vi "CAN Jaguar Set PID.vi"(0 "CAN Jaguar Ref":T1={"Device Number"=0, "Control Mode"=enum."Percent VBus", "Inverted"=FALSE, "Semaphore"=refnum, "Max Vout"=12.0, "DevStatus"={"status"=FALSE, "code"=0, "source"=""}}, 5 "P":dbl, 7 "I":dbl, 9 "D":dbl, 11 "error in (no error)":errorcluster) -> (4 "CAN Jaguar Ref Out":T1={"Device Number"=0, "Control Mode"=enum."Percent VBus", "Inverted"=FALSE, "Semaphore"=refnum, "Max Vout"=12.0, "DevStatus"={"status"=FALSE, "code"=0, "source"=""}}, 15 "error out":errorcluster)   [LabVIEW 2009, in "CAN.lvlib"]
uses:
  CAN.lvlib
  SubVIs/CAN Motor Message IDs.ctl
  SubVIs/CAN Jaguar Control Mode.ctl
  SubVIs/CAN Jaguar Ref.ctl
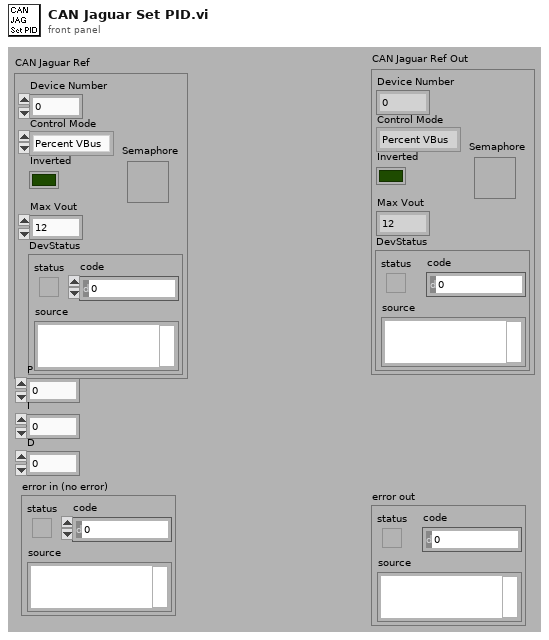
[diagram p1: front panel]
types:
  T1 = typedef "CAN.lvlib/CAN Jaguar Ref.ctl" = cluster{"Device Number":u8, "Control Mode":T2, "Inverted":bool, "Semaphore":T3, "Max Vout":dbl, "DevStatus":errorcluster}
  T2 = typedef "CAN.lvlib/CAN Jaguar Control Mode.ctl" = enum16{"Percent VBus", "Speed", "Position", "Current"}
  T3 = typedef "Semaphore RefNum" = refnum<k1>
  T4 = enum16{"big-endian, network order", "native, host order", "little-endian"}
  T5 = typedef "CAN.lvlib/CAN Motor Message IDs.ctl" = u32
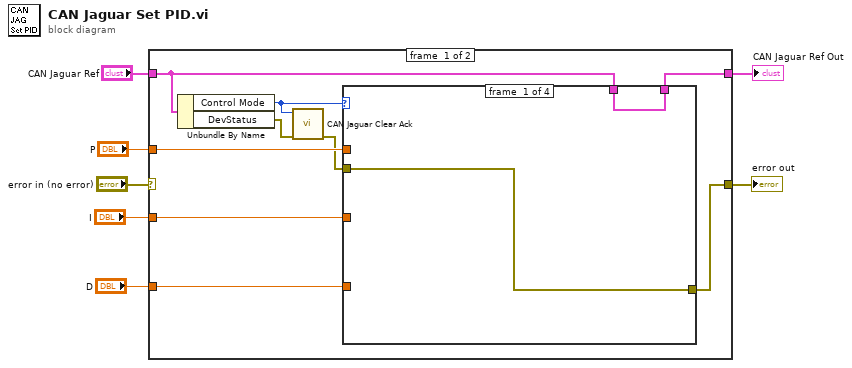
[diagram p0: block diagram]
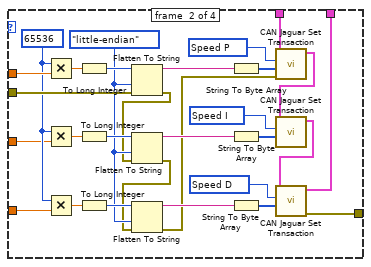
[diagram p2: hidden frame]
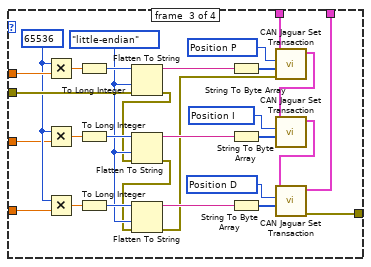
[diagram p3: hidden frame]
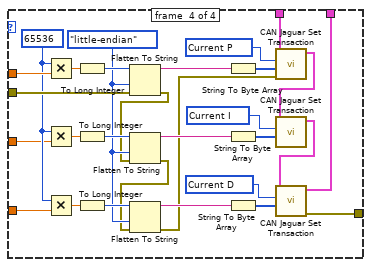
[diagram p4: hidden frame]
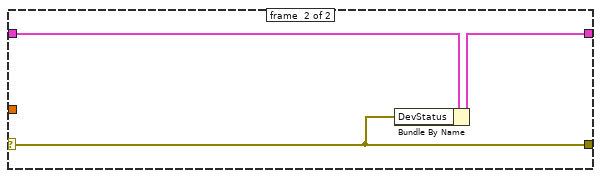
[diagram p5: hidden frame]
diagram:
  n1 = case shown="No Error" "error in (no error)" {
    selector: "error in (no error)" -> [_ w106]
    tunnel: [w13 w106] -> w7
    tunnel: [w8 w107] -> w5
    tunnel: "CAN Jaguar Ref" -> [w9 w108]
    tunnel: "P" -> [w16 _]
    tunnel: "D" -> [w15 _]
    tunnel: "I" -> [w14 _]
    frame #0 {
      n2 = Unbundle By Name(w9) -> ("Control Mode"=w10:T2, "DevStatus"=w12:errorcluster)
      n3 = call "CAN Jaguar Clear Ack.vi"("DevStatus"=w12, "Device Number"=w10) -> ("error out"=w11:errorcluster)  [unwired: 9 out]
      n4 = case shown="\"Speed\"" w10 {
        tunnel: w11 -> [w18 w46 w75 w104]
        tunnel: w16 -> [_ w44 w73 w102]
        tunnel: w15 -> [_ w34 w63 w92]
        tunnel: w14 -> [_ w33 w62 w91]
        tunnel: [w18 w20 w49 w77] -> w13
        tunnel: w9 -> [w17 w29 w56 w86]
        tunnel: [w17 w19 w48 w82] -> w8
        frame #0 {
        }
        frame #1 {
          w36 = T4."little-endian" ("byte order (0:big-endian, network order)")
          w30 = T5 33686848 items=["Volt Enable"=33685504, "Volt Disable"=33685568, "Volt Set"=33685632, "Volt Set Ramp"=33685696, "Speed Enable"=33686528, "Speed Disable"=33686592, "Speed Set"=33686656, "Speed P"=33686720, "Speed I"=33686784, "Speed D"=33686848, "Speed Ref"=33686912, "Position Enable"=33688576, "Position Disable"=33688640, "Position Set"=33688704, "Position P"=33688768, "Position I"=33688832, "Position D"=33688896, "Position Ref"=33688960, "Current Enable"=33689600, "Current Disable"=33689664, "Current Set"=33689728, "Current P"=33689792, "Current I"=33689856, "Current D"=33689920, "Status VOut"=33690624, "Status VBus"=33690688, "Status Current"=33690752, "Status Temp"=33690816, "Status Position"=33690880, "Status Speed"=33690944, "Status Limit"=33691008, "Status Fault"=33691072, "Status Power"=33691136, "Config Num Brushes"=33692672, "Config Encoder Lines"=33692736, "Config Pot Turns"=33692800, "Config Brake Coast"=33692864, "Config Limit Mode"=33692928, "Config Limit Fwd"=33692992, "Config Limit Rev"=33693056, "Config Max VOut"=33693120, "Config Fault Time"=33693184, "Motor Ack"=33693696] ("CAN Motor Message IDs")
          w24 = T5 33686784 items=["Volt Enable"=33685504, "Volt Disable"=33685568, "Volt Set"=33685632, "Volt Set Ramp"=33685696, "Speed Enable"=33686528, "Speed Disable"=33686592, "Speed Set"=33686656, "Speed P"=33686720, "Speed I"=33686784, "Speed D"=33686848, "Speed Ref"=33686912, "Position Enable"=33688576, "Position Disable"=33688640, "Position Set"=33688704, "Position P"=33688768, "Position I"=33688832, "Position D"=33688896, "Position Ref"=33688960, "Current Enable"=33689600, "Current Disable"=33689664, "Current Set"=33689728, "Current P"=33689792, "Current I"=33689856, "Current D"=33689920, "Status VOut"=33690624, "Status VBus"=33690688, "Status Current"=33690752, "Status Temp"=33690816, "Status Position"=33690880, "Status Speed"=33690944, "Status Limit"=33691008, "Status Fault"=33691072, "Status Power"=33691136, "Config Num Brushes"=33692672, "Config Encoder Lines"=33692736, "Config Pot Turns"=33692800, "Config Brake Coast"=33692864, "Config Limit Mode"=33692928, "Config Limit Fwd"=33692992, "Config Limit Rev"=33693056, "Config Max VOut"=33693120, "Config Fault Time"=33693184, "Motor Ack"=33693696] ("CAN Motor Message IDs")
          w35 = 65536
          w27 = T5 33686720 items=["Volt Enable"=33685504, "Volt Disable"=33685568, "Volt Set"=33685632, "Volt Set Ramp"=33685696, "Speed Enable"=33686528, "Speed Disable"=33686592, "Speed Set"=33686656, "Speed P"=33686720, "Speed I"=33686784, "Speed D"=33686848, "Speed Ref"=33686912, "Position Enable"=33688576, "Position Disable"=33688640, "Position Set"=33688704, "Position P"=33688768, "Position I"=33688832, "Position D"=33688896, "Position Ref"=33688960, "Current Enable"=33689600, "Current Disable"=33689664, "Current Set"=33689728, "Current P"=33689792, "Current I"=33689856, "Current D"=33689920, "Status VOut"=33690624, "Status VBus"=33690688, "Status Current"=33690752, "Status Temp"=33690816, "Status Position"=33690880, "Status Speed"=33690944, "Status Limit"=33691008, "Status Fault"=33691072, "Status Power"=33691136, "Config Num Brushes"=33692672, "Config Encoder Lines"=33692736, "Config Pot Turns"=33692800, "Config Brake Coast"=33692864, "Config Limit Mode"=33692928, "Config Limit Fwd"=33692992, "Config Limit Rev"=33693056, "Config Max VOut"=33693120, "Config Fault Time"=33693184, "Motor Ack"=33693696] ("CAN Motor Message IDs")
          n5 = Multiply(x=w35, y=w44) -> (x*y=w45:dbl)
          n6 = Multiply(x=w35, y=w33) -> (x*y=w43:dbl)
          n7 = Multiply(x=w35, y=w34) -> (x*y=w40:dbl)
          n8 = To Long Integer(number=w45) -> (32bit integer=w47:i32)
          n9 = To Long Integer(number=w43) -> (32bit integer=w42:i32)
          n10 = To Long Integer(number=w40) -> (32bit integer=w41:i32)
          n11 = Flatten To String(anything=w47, byte order (0:big-endian, network order)=w36, error in (no error)=w46) -> (data string=w39:string, error out=w32:errorcluster)  [unwired: 2 out]
          n12 = Flatten To String(anything=w42, byte order (0:big-endian, network order)=w36, error in (no error)=w32) -> (data string=w38:string, error out=w31:errorcluster)  [unwired: 2 out]
          n13 = Flatten To String(anything=w41, byte order (0:big-endian, network order)=w36, error in (no error)=w31) -> (data string=w37:string, error out=w28:errorcluster)  [unwired: 2 out]
          n14 = String To Byte Array(string=w39) -> (unsigned byte array=w26:u8[])
          n15 = String To Byte Array(string=w38) -> (unsigned byte array=w25:u8[])
          n16 = String To Byte Array(string=w37) -> (unsigned byte array=w22:u8[])
          n17 = call "CAN Jaguar Set Transaction.vi"("error in"=w28, "Data"=w26, "Message ID"=w27, "CAN Jaguar Ref"=w29) -> ("CAN Jaguar Ref Out"=w23:T1)  [unwired: 7 out]
          n18 = call "CAN Jaguar Set Transaction.vi"("Data"=w25, "Message ID"=w24, "CAN Jaguar Ref"=w23) -> ("CAN Jaguar Ref Out"=w21:T1)  [unwired: 1 in, 7 out]
          n19 = call "CAN Jaguar Set Transaction.vi"("Data"=w22, "Message ID"=w30, "CAN Jaguar Ref"=w21) -> ("error out"=w20:errorcluster, "CAN Jaguar Ref Out"=w19:T1)  [unwired: 1 in, 6 out]
        }
        frame #2 {
          w65 = T4."little-endian" ("byte order (0:big-endian, network order)")
          w53 = T5 33688896 items=["Volt Enable"=33685504, "Volt Disable"=33685568, "Volt Set"=33685632, "Volt Set Ramp"=33685696, "Speed Enable"=33686528, "Speed Disable"=33686592, "Speed Set"=33686656, "Speed P"=33686720, "Speed I"=33686784, "Speed D"=33686848, "Speed Ref"=33686912, "Position Enable"=33688576, "Position Disable"=33688640, "Position Set"=33688704, "Position P"=33688768, "Position I"=33688832, "Position D"=33688896, "Position Ref"=33688960, "Current Enable"=33689600, "Current Disable"=33689664, "Current Set"=33689728, "Current P"=33689792, "Current I"=33689856, "Current D"=33689920, "Status VOut"=33690624, "Status VBus"=33690688, "Status Current"=33690752, "Status Temp"=33690816, "Status Position"=33690880, "Status Speed"=33690944, "Status Limit"=33691008, "Status Fault"=33691072, "Status Power"=33691136, "Config Num Brushes"=33692672, "Config Encoder Lines"=33692736, "Config Pot Turns"=33692800, "Config Brake Coast"=33692864, "Config Limit Mode"=33692928, "Config Limit Fwd"=33692992, "Config Limit Rev"=33693056, "Config Max VOut"=33693120, "Config Fault Time"=33693184, "Motor Ack"=33693696] ("CAN Motor Message IDs")
          w52 = T5 33688832 items=["Volt Enable"=33685504, "Volt Disable"=33685568, "Volt Set"=33685632, "Volt Set Ramp"=33685696, "Speed Enable"=33686528, "Speed Disable"=33686592, "Speed Set"=33686656, "Speed P"=33686720, "Speed I"=33686784, "Speed D"=33686848, "Speed Ref"=33686912, "Position Enable"=33688576, "Position Disable"=33688640, "Position Set"=33688704, "Position P"=33688768, "Position I"=33688832, "Position D"=33688896, "Position Ref"=33688960, "Current Enable"=33689600, "Current Disable"=33689664, "Current Set"=33689728, "Current P"=33689792, "Current I"=33689856, "Current D"=33689920, "Status VOut"=33690624, "Status VBus"=33690688, "Status Current"=33690752, "Status Temp"=33690816, "Status Position"=33690880, "Status Speed"=33690944, "Status Limit"=33691008, "Status Fault"=33691072, "Status Power"=33691136, "Config Num Brushes"=33692672, "Config Encoder Lines"=33692736, "Config Pot Turns"=33692800, "Config Brake Coast"=33692864, "Config Limit Mode"=33692928, "Config Limit Fwd"=33692992, "Config Limit Rev"=33693056, "Config Max VOut"=33693120, "Config Fault Time"=33693184, "Motor Ack"=33693696] ("CAN Motor Message IDs")
          w64 = 65536
          w57 = T5 33688768 items=["Volt Enable"=33685504, "Volt Disable"=33685568, "Volt Set"=33685632, "Volt Set Ramp"=33685696, "Speed Enable"=33686528, "Speed Disable"=33686592, "Speed Set"=33686656, "Speed P"=33686720, "Speed I"=33686784, "Speed D"=33686848, "Speed Ref"=33686912, "Position Enable"=33688576, "Position Disable"=33688640, "Position Set"=33688704, "Position P"=33688768, "Position I"=33688832, "Position D"=33688896, "Position Ref"=33688960, "Current Enable"=33689600, "Current Disable"=33689664, "Current Set"=33689728, "Current P"=33689792, "Current I"=33689856, "Current D"=33689920, "Status VOut"=33690624, "Status VBus"=33690688, "Status Current"=33690752, "Status Temp"=33690816, "Status Position"=33690880, "Status Speed"=33690944, "Status Limit"=33691008, "Status Fault"=33691072, "Status Power"=33691136, "Config Num Brushes"=33692672, "Config Encoder Lines"=33692736, "Config Pot Turns"=33692800, "Config Brake Coast"=33692864, "Config Limit Mode"=33692928, "Config Limit Fwd"=33692992, "Config Limit Rev"=33693056, "Config Max VOut"=33693120, "Config Fault Time"=33693184, "Motor Ack"=33693696] ("CAN Motor Message IDs")
          n20 = Multiply(x=w64, y=w73) -> (x*y=w74:dbl)
          n21 = Multiply(x=w64, y=w62) -> (x*y=w72:dbl)
          n22 = Multiply(x=w64, y=w63) -> (x*y=w69:dbl)
          n23 = To Long Integer(number=w74) -> (32bit integer=w76:i32)
          n24 = To Long Integer(number=w72) -> (32bit integer=w71:i32)
          n25 = To Long Integer(number=w69) -> (32bit integer=w70:i32)
          n26 = Flatten To String(anything=w76, byte order (0:big-endian, network order)=w65, error in (no error)=w75) -> (data string=w68:string, error out=w61:errorcluster)  [unwired: 2 out]
          n27 = Flatten To String(anything=w71, byte order (0:big-endian, network order)=w65, error in (no error)=w61) -> (data string=w67:string, error out=w60:errorcluster)  [unwired: 2 out]
          n28 = Flatten To String(anything=w70, byte order (0:big-endian, network order)=w65, error in (no error)=w60) -> (data string=w66:string, error out=w58:errorcluster)  [unwired: 2 out]
          n29 = String To Byte Array(string=w68) -> (unsigned byte array=w59:u8[])
          n30 = String To Byte Array(string=w67) -> (unsigned byte array=w55:u8[])
          n31 = String To Byte Array(string=w66) -> (unsigned byte array=w54:u8[])
          n32 = call "CAN Jaguar Set Transaction.vi"("error in"=w58, "Data"=w59, "Message ID"=w57, "CAN Jaguar Ref"=w56) -> ("CAN Jaguar Ref Out"=w51:T1)  [unwired: 7 out]
          n33 = call "CAN Jaguar Set Transaction.vi"("Data"=w55, "Message ID"=w52, "CAN Jaguar Ref"=w51) -> ("CAN Jaguar Ref Out"=w50:T1)  [unwired: 1 in, 7 out]
          n34 = call "CAN Jaguar Set Transaction.vi"("Data"=w54, "Message ID"=w53, "CAN Jaguar Ref"=w50) -> ("error out"=w49:errorcluster, "CAN Jaguar Ref Out"=w48:T1)  [unwired: 1 in, 6 out]
        }
        frame #3 {
          w94 = T4."little-endian" ("byte order (0:big-endian, network order)")
          w81 = T5 33689920 items=["Volt Enable"=33685504, "Volt Disable"=33685568, "Volt Set"=33685632, "Volt Set Ramp"=33685696, "Speed Enable"=33686528, "Speed Disable"=33686592, "Speed Set"=33686656, "Speed P"=33686720, "Speed I"=33686784, "Speed D"=33686848, "Speed Ref"=33686912, "Position Enable"=33688576, "Position Disable"=33688640, "Position Set"=33688704, "Position P"=33688768, "Position I"=33688832, "Position D"=33688896, "Position Ref"=33688960, "Current Enable"=33689600, "Current Disable"=33689664, "Current Set"=33689728, "Current P"=33689792, "Current I"=33689856, "Current D"=33689920, "Status VOut"=33690624, "Status VBus"=33690688, "Status Current"=33690752, "Status Temp"=33690816, "Status Position"=33690880, "Status Speed"=33690944, "Status Limit"=33691008, "Status Fault"=33691072, "Status Power"=33691136, "Config Num Brushes"=33692672, "Config Encoder Lines"=33692736, "Config Pot Turns"=33692800, "Config Brake Coast"=33692864, "Config Limit Mode"=33692928, "Config Limit Fwd"=33692992, "Config Limit Rev"=33693056, "Config Max VOut"=33693120, "Config Fault Time"=33693184, "Motor Ack"=33693696] ("CAN Motor Message IDs")
          w80 = T5 33689856 items=["Volt Enable"=33685504, "Volt Disable"=33685568, "Volt Set"=33685632, "Volt Set Ramp"=33685696, "Speed Enable"=33686528, "Speed Disable"=33686592, "Speed Set"=33686656, "Speed P"=33686720, "Speed I"=33686784, "Speed D"=33686848, "Speed Ref"=33686912, "Position Enable"=33688576, "Position Disable"=33688640, "Position Set"=33688704, "Position P"=33688768, "Position I"=33688832, "Position D"=33688896, "Position Ref"=33688960, "Current Enable"=33689600, "Current Disable"=33689664, "Current Set"=33689728, "Current P"=33689792, "Current I"=33689856, "Current D"=33689920, "Status VOut"=33690624, "Status VBus"=33690688, "Status Current"=33690752, "Status Temp"=33690816, "Status Position"=33690880, "Status Speed"=33690944, "Status Limit"=33691008, "Status Fault"=33691072, "Status Power"=33691136, "Config Num Brushes"=33692672, "Config Encoder Lines"=33692736, "Config Pot Turns"=33692800, "Config Brake Coast"=33692864, "Config Limit Mode"=33692928, "Config Limit Fwd"=33692992, "Config Limit Rev"=33693056, "Config Max VOut"=33693120, "Config Fault Time"=33693184, "Motor Ack"=33693696] ("CAN Motor Message IDs")
          w93 = 65536
          w85 = T5 33689792 items=["Volt Enable"=33685504, "Volt Disable"=33685568, "Volt Set"=33685632, "Volt Set Ramp"=33685696, "Speed Enable"=33686528, "Speed Disable"=33686592, "Speed Set"=33686656, "Speed P"=33686720, "Speed I"=33686784, "Speed D"=33686848, "Speed Ref"=33686912, "Position Enable"=33688576, "Position Disable"=33688640, "Position Set"=33688704, "Position P"=33688768, "Position I"=33688832, "Position D"=33688896, "Position Ref"=33688960, "Current Enable"=33689600, "Current Disable"=33689664, "Current Set"=33689728, "Current P"=33689792, "Current I"=33689856, "Current D"=33689920, "Status VOut"=33690624, "Status VBus"=33690688, "Status Current"=33690752, "Status Temp"=33690816, "Status Position"=33690880, "Status Speed"=33690944, "Status Limit"=33691008, "Status Fault"=33691072, "Status Power"=33691136, "Config Num Brushes"=33692672, "Config Encoder Lines"=33692736, "Config Pot Turns"=33692800, "Config Brake Coast"=33692864, "Config Limit Mode"=33692928, "Config Limit Fwd"=33692992, "Config Limit Rev"=33693056, "Config Max VOut"=33693120, "Config Fault Time"=33693184, "Motor Ack"=33693696] ("CAN Motor Message IDs")
          n35 = Multiply(x=w93, y=w102) -> (x*y=w103:dbl)
          n36 = Multiply(x=w93, y=w91) -> (x*y=w101:dbl)
          n37 = Multiply(x=w93, y=w92) -> (x*y=w98:dbl)
          n38 = To Long Integer(number=w103) -> (32bit integer=w105:i32)
          n39 = To Long Integer(number=w101) -> (32bit integer=w100:i32)
          n40 = To Long Integer(number=w98) -> (32bit integer=w99:i32)
          n41 = Flatten To String(anything=w105, byte order (0:big-endian, network order)=w94, error in (no error)=w104) -> (data string=w97:string, error out=w90:errorcluster)  [unwired: 2 out]
          n42 = Flatten To String(anything=w100, byte order (0:big-endian, network order)=w94, error in (no error)=w90) -> (data string=w96:string, error out=w89:errorcluster)  [unwired: 2 out]
          n43 = Flatten To String(anything=w99, byte order (0:big-endian, network order)=w94, error in (no error)=w89) -> (data string=w95:string, error out=w88:errorcluster)  [unwired: 2 out]
          n44 = String To Byte Array(string=w97) -> (unsigned byte array=w87:u8[])
          n45 = String To Byte Array(string=w96) -> (unsigned byte array=w84:u8[])
          n46 = String To Byte Array(string=w95) -> (unsigned byte array=w83:u8[])
          n47 = call "CAN Jaguar Set Transaction.vi"("error in"=w88, "Data"=w87, "Message ID"=w85, "CAN Jaguar Ref"=w86) -> ("CAN Jaguar Ref Out"=w79:T1)  [unwired: 7 out]
          n48 = call "CAN Jaguar Set Transaction.vi"("Data"=w84, "Message ID"=w80, "CAN Jaguar Ref"=w79) -> ("CAN Jaguar Ref Out"=w78:T1)  [unwired: 1 in, 7 out]
          n49 = call "CAN Jaguar Set Transaction.vi"("Data"=w83, "Message ID"=w81, "CAN Jaguar Ref"=w78) -> ("error out"=w77:errorcluster, "CAN Jaguar Ref Out"=w82:T1)  [unwired: 1 in, 6 out]
        }
      }
    }
    frame #1 {
      n50 = Bundle By Name(cluster=w108, "DevStatus"=w106) -> (w107:T1)
    }
  }
  "CAN Jaguar Ref Out" <- w5
  "error out" <- w7
